vi "read from hannes.vi"() -> ()   [LabVIEW 2016]
panel:
  out "Array":dbl[][](array[numeric])
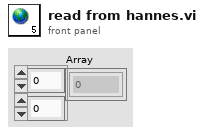
[diagram p1: front panel]
diagram:
